vi "Ej_11_Nodos_de_Propiedad.vi"() -> ()   [LabVIEW 2021]
panel:
  in  "Posición Horizontal":dbl(slide) scale=0.0..400.0
  out "Cadena Caracteres":string
  in  "Boolean":bool
  in  "Posición Vertical":dbl(slide) scale=0.0..300.0
  in  "Deshabilitar":bool
  in  "Límite":dbl
  in  "stop":bool
  out "Tank":dbl(slide) scale=0.0..10.0
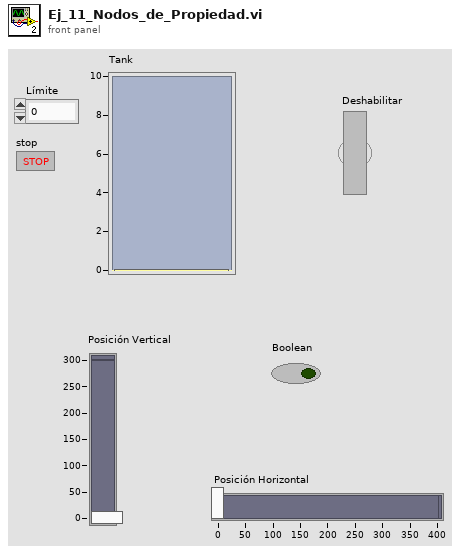
[diagram p1: front panel]
types:
  T1 = cluster{"Posición Vertical":dbl, "Posición Horizontal":dbl}
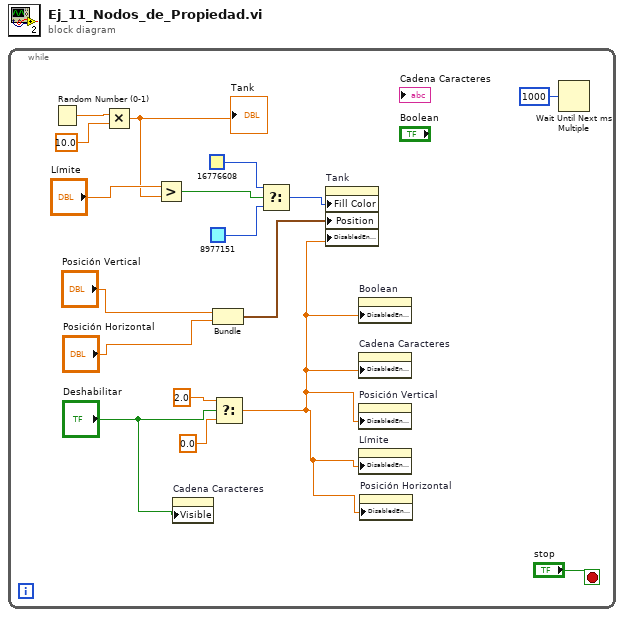
[diagram p0: block diagram]
diagram:
  n1 = while {
    stop <- "stop" stop-if-true
    n2 = Random Number (0-1)() -> (number: 0 to 1=w16:dbl)
    n3 = Multiply(x=w16, y=10.0) -> (x*y=w13:dbl)
    "Tank" <- w13
    n4 = Greater?(x="Límite", y=w13) -> (0:w12:bool)
    n5 = property on="Cadena Caracteres" class="Str"("Visible"="Deshabilitar") -> ()  [unwired: 2 in, 2 out]
    n6 = Bundle("Posición Vertical"="Posición Vertical", "Posición Horizontal"="Posición Horizontal") -> (w5:T1)  [unwired: 1 in]
    n7 = Select(t=2.0, s="Deshabilitar", f=0.0) -> (s? t:f=w2:dbl)
    n8 = Select(t=u32 16776608, s=w12, f=u32 8977151) -> (s? t:f=w8:u32)
    n9 = property on="Tank" class="Slide (strict)"("Fill Color"=w8, "Position"=w5, "DisabledEnum"=w2) -> ()  [unwired: 2 in, 2 out]
    n10 = property on="Boolean" class="Bool (strict)"("DisabledEnum"=w2) -> ()  [unwired: 2 in, 2 out]
    n11 = property on="Cadena Caracteres" class="Str"("DisabledEnum"=w2) -> ()  [unwired: 2 in, 2 out]
    n12 = property on="Posición Vertical" class="Slide (strict)"("DisabledEnum"=w2) -> ()  [unwired: 2 in, 2 out]
    n13 = property on="Límite" class="DigNum (strict)"("DisabledEnum"=w2) -> ()  [unwired: 2 in, 2 out]
    n14 = property on="Posición Horizontal" class="Slide (strict)"("DisabledEnum"=w2) -> ()  [unwired: 2 in, 2 out]
    n15 = Wait Until Next ms Multiple(millisecond multiple=u32 1000) -> ()  [unwired: 1 out]
  }
